vi "Waveform_Append and Resize Allocated.vi"(8 "Error":errorcluster, 9 "Append":T1, 11 "Waveform":T1) -> (0 "Error Out":errorcluster, 3 "Waveform Out":T1, 5 "Offset Out":i32)   [LabVIEW 2016]
uses:
  Universal Controls/Waveform_Data.ctl
  Universal Controls/Read Write Button.ctl
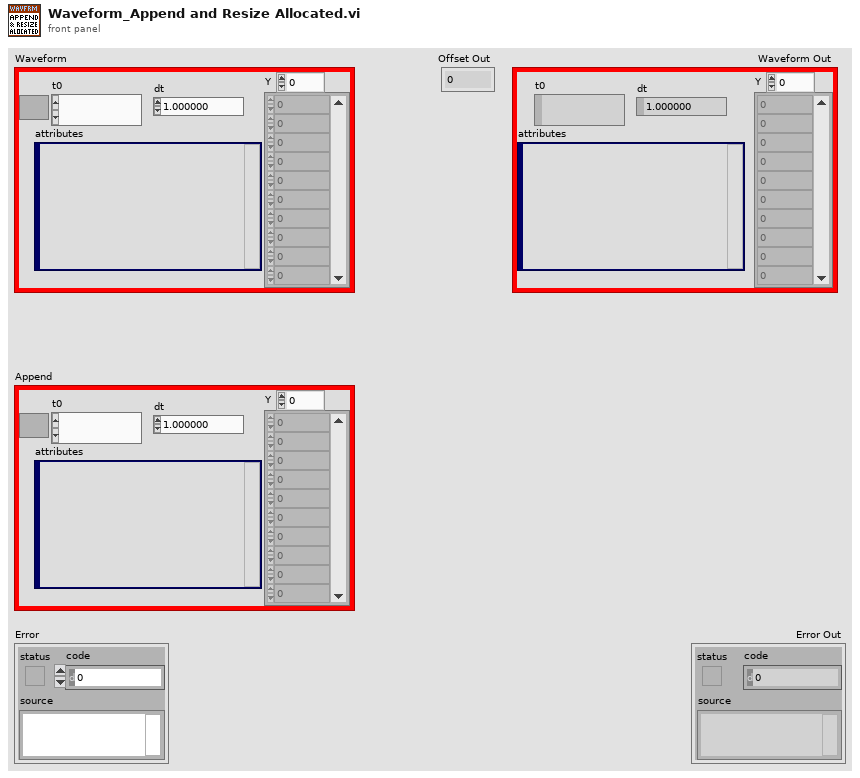
[diagram p1: front panel]
types:
  T1 = typedef "Waveform_Data.ctl" = waveform(dbl)
  T2 = typedef "Read Write Button.ctl" = bool
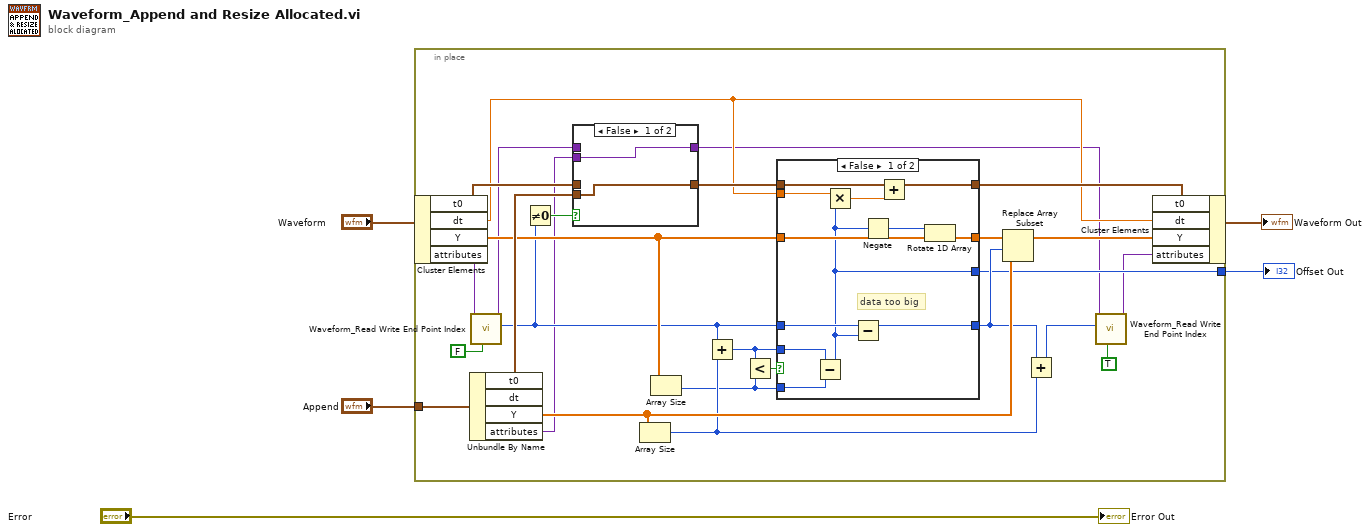
[diagram p0: block diagram]
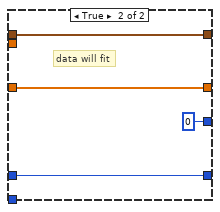
[diagram p3: hidden frame]
diagram:
  n1 = in-place {
    in-place-border: "Append" -> [w30]
    in-place-border: [w21] -> w3
    n2 = in-place-cluster #1("Waveform") -> ("t0"=w31:timestamp, "dt"=w10:dbl, "Y"=w27:dbl[], "attributes"=w16:variant)
    n3 = Unbundle By Name(w30) -> ("t0"=w29:timestamp, "Y"=w25:dbl[], "attributes"=w6:variant)  [unwired: 1 out]
    n4 = call "Waveform_Read Write End Point Index.vi"("Read(f)\nWrite(t)"=T2 FALSE ("Read(f)\nWrite(t)"), "Waveform Atributes"=w16) -> ("End Point Out"=w12:i32, "Waveform Atributes Out"=w9:variant)  [unwired: 7 in, 1 out]
    n5 = Not Equal To 0?(x=w12) -> (x != 0?=w7:bool)
    n6 = case shown="False" w7 {
      tunnel: w31 -> [_ w35]
      tunnel: w29 -> [w33 _]
      tunnel: [w33 w35] -> w20
      tunnel: w9 -> [_ w34]
      tunnel: [w32 w34] -> w8
      tunnel: w6 -> [w32 _]
      frame False {
      }
      frame True {
      }
    }
    n7 = Array Size(array=w25) -> (size(s)=w23:i32)
    n8 = Array Size(array=w27) -> (size(s)=w17:i32)
    n9 = Add(x=w12, y=w23) -> (x+y=w18:i32)
    n10 = Less?(x=w18, y=w17) -> (x < y?=w28:bool)
    n11 = case shown="False" w28 {
      tunnel: w18 -> [w46 _]
      tunnel: w17 -> [w47 _]
      tunnel: w12 -> [w44 w51]
      tunnel: w27 -> [w45 w50]
      tunnel: [w43 w50] -> w26
      tunnel: [w42 w51] -> w22
      tunnel: [w40 0] -> w21
      tunnel: w20 -> [w41 w49]
      tunnel: [w38 w49] -> w19
      tunnel: w10 -> [w39 _]
      frame False {
        # "data too big"
        n12 = Subtract(x=w46, y=w47) -> (x-y=w40:i32)
        n13 = Multiply(x=w39, y=w40) -> (x*y=w37:dbl)
        n14 = Subtract(x=w44, y=w40) -> (x-y=w42:i32)
        n15 = Negate(x=w40) -> (-x=w36:i32)
        n16 = Add(x=w41, y=w37) -> (x+y=w38:timestamp)
        n17 = Rotate 1D Array(1:w45, 2:w36) -> (0:w43:dbl[])
      }
      frame True {
        # "data will fit"
      }
    }
    n18 = Replace Array Subset(array=w26, new element=w25, index=w22) -> (w24:dbl[])
    n19 = Add(x=w22, y=w23) -> (x+y=w11:i32)
    n20 = call "Waveform_Read Write End Point Index.vi"("Read(f)\nWrite(t)"=T2 TRUE ("Read(f)\nWrite(t)"), "End Point"=w11, "Waveform Atributes"=w8) -> ("Waveform Atributes Out"=w15:variant)  [unwired: 6 in, 2 out]
    n21 = in-place-cluster #1("t0"=w19, "dt"=w10, "Y"=w24, "attributes"=w15) -> (→"Waveform Out":T1)
  }
  "Offset Out" <- w3
  "Error Out" <- "Error"
